vi "pll_proba_diag.vi"(0 "all rows":dbl[][](array[numeric])=array100002x3[300006 elements] format="%0.5f", 1 "Second":bool, 5 "Resolution":dbl, 7 "t_ref":dbl[](array[numeric]), 9 "dt":dbl, 11 "Error In":errorcluster) -> (3 "average":dbl=2.3596690204414683, 4 "XY Graph":cluster{"all rows":dbl[], "all rows":dbl[]}[](graph), 6 "Waveform Graph":cluster{"f0":dbl, "df":dbl, "magnitude":dbl[]}(graph), 8 "time":dbl[](array[numeric]), 10 "Waveform Graph 2":cluster{"f0":dbl, "df":dbl, "magnitude":dbl[]}(graph), 13 "PLL_sine":dbl[](array[numeric]), 14 "PLL_cosine":dbl[](array[numeric]), 15 "Error Out":errorcluster)   [LabVIEW 2013]
uses:
  <vilib>/Utility/file.llb/Read From Spreadsheet File (DBL).vi
  <vilib>/Utility/file.llb/Write To Spreadsheet File (DBL).vi
  <vilib>/express/express analysis/Spectral/Block/exnSpectralBlock spectral measurements RMS poly.vi
  <vilib>/express/express analysis/Spectral/Block/exnSpectralBlock spectral measurements RMS WFM.vi
  <vilib>/express/express analysis/Spectral/XNode/ExpressSpectralMeasurementsBlockNode.xnode
panel:
  out "sin(x)":dbl[](array[numeric])
  out "Array":dbl[](array[numeric])
  out "file path (use dialog)":path=path "C:/Users/Orban Anges/Desktop/DIAG_Prog_v2/temp.txt"
  out "XY Graph 2":cluster{"all rows":dbl[], "all rows":dbl[]}[](graph)
  out "t_i-1":dbl
  out "t_i":dbl
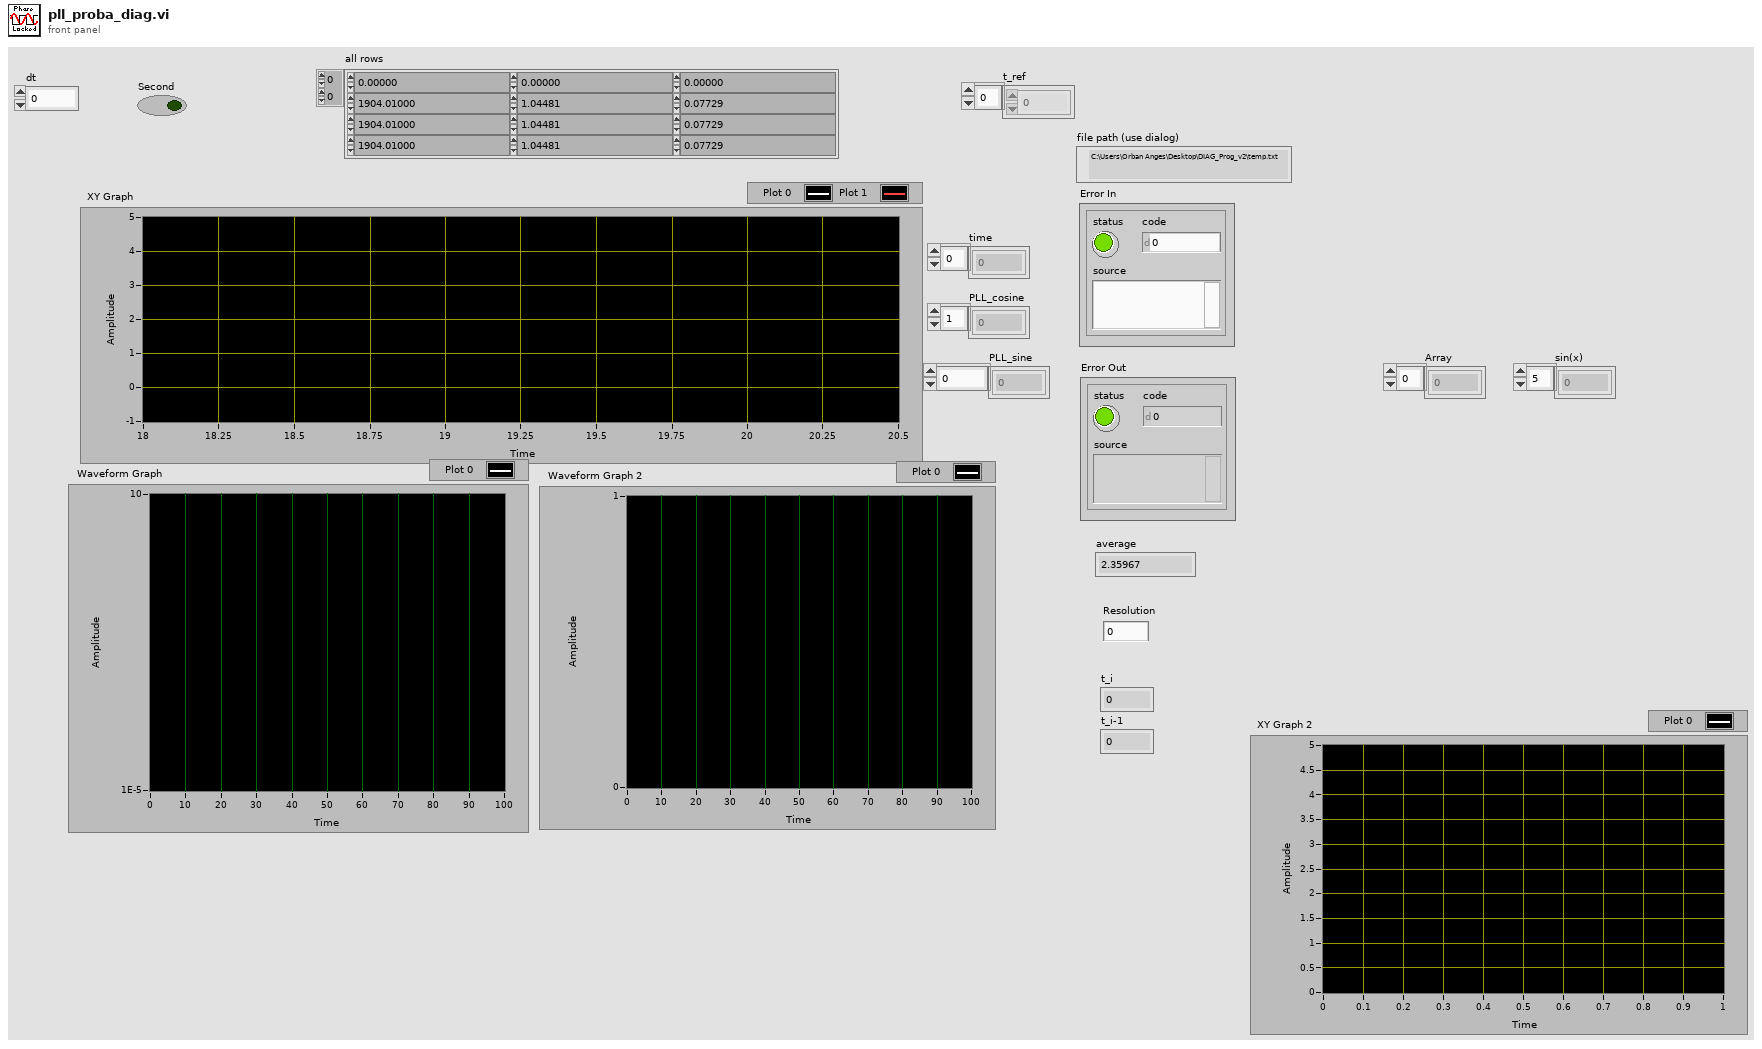
[diagram p1: front panel]
types:
  T1 = enum16{"open", "replace", "create", "open or create", "replace or create", "replace or create with confirmation"}
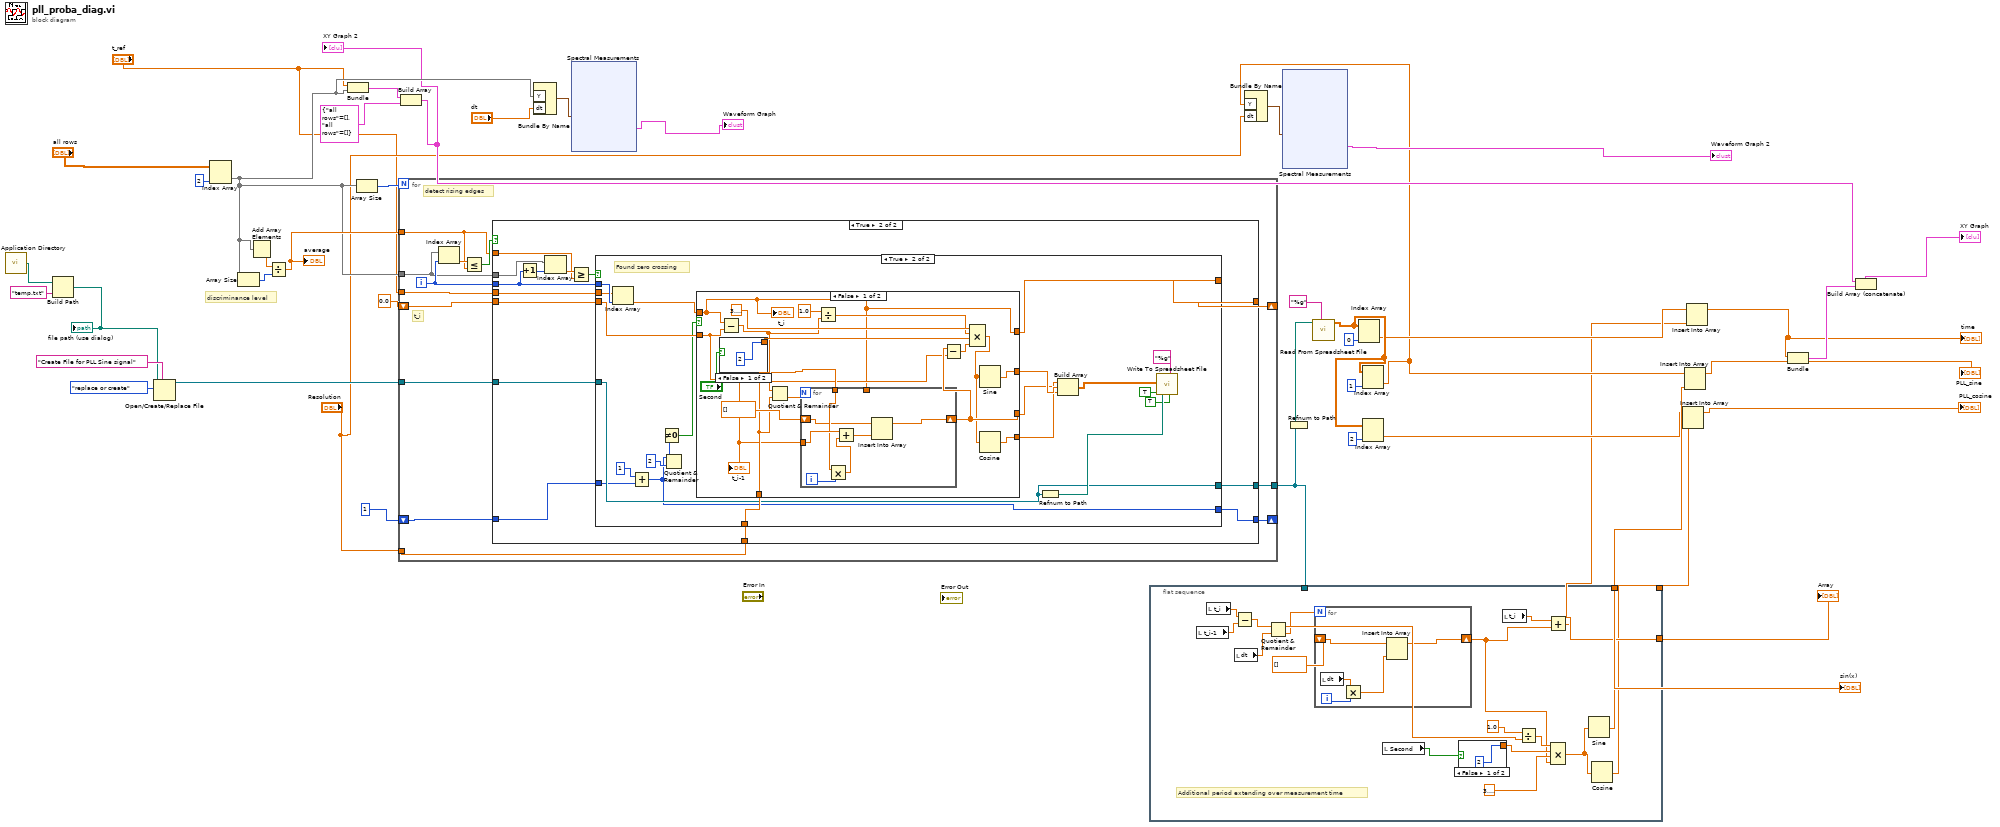
[diagram p0: block diagram]
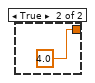
[diagram p2: hidden frame]
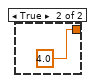
[diagram p5: hidden frame]
diagram:
  # "discriminance level"
  n1 = call <vilib>:"Application Directory.vi"() -> ("Application Directory"=w14:path)
  n2 = Build Path(base path=w14, name or relative path="temp.txt") -> (appended path=w12:path)
  "file path (use dialog)" <- w12
  n3 = Open/Create/Replace File(file path (use dialog)=w12, prompt="Create File for PLL Sine signal", operation (0:open)=T1."replace or create") -> (refnum out=w34:refnum<file>)  [unwired: 3 in, 2 out]
  n4 = Index Array(array="all rows", index (col)=2 ("disabled index (col)")) -> (element=w27:dbl[])  [unwired: 1 in]
  n5 = Array Size(array=w27) -> (size(s)=w40:i32)
  n6 = Add Array Elements(numeric array=w27) -> (sum=w41:dbl)
  n7 = Divide(x=w41, y=w40) -> (x/y=w39:dbl)
  "average" <- w39
  n8 = Bundle("t_ref"="t_ref", "all rows"=w27) -> (w21:cluster{"t_ref":dbl[], "all rows":dbl[]})  [unwired: 1 in]
  n9 = Array Size(array=w27) -> (size(s)=w38:i32)
  n10 = for {
    N: w38 -> [_]
    tunnel: w27 -> [w54]
    tunnel: w39 -> [w52]
    tunnel: "t_ref" -> [w51]
    shift-right: [w50] -> _
    shift-left: 0.0 -> [w44]
    tunnel: "Resolution" -> [w49]
    tunnel: w34 -> [w48]
    tunnel: [w47] -> w1
    shift-right: [w45] -> _
    shift-left: 1 -> [w46]
    i -> [w55]
    # "t_i"
    # "detect rising edges"
    n11 = Index Array(array=w54, index=w55) -> (element=w53:dbl)
    n12 = Less Or Equal?(x=w53, y=w52) -> (x <= y?=w56:bool)
    n13 = case shown="True" w56 {
      tunnel: w55 -> [_ w67]
      tunnel: w54 -> [_ w73]
      tunnel: w52 -> [_ w69]
      tunnel: w51 -> [_ w68]
      tunnel: [w59 w66] -> w50
      tunnel: w44 -> [w59 w60]
      tunnel: w49 -> [_ w65]
      tunnel: w48 -> [w58 w64]
      tunnel: [w58 w63] -> w47
      tunnel: w46 -> [w57 w62]
      tunnel: [w57 w61] -> w45
      frame False {
      }
      frame True {
        n14 = Increment(x=w67) -> (x+1=w72:i32)
        n15 = Index Array(array=w73, index=w72) -> (element=w70:dbl)
        n16 = Greater Or Equal?(x=w70, y=w69) -> (x >= y?=w71:bool)
        n17 = case shown="True" w71 {
          tunnel: w68 -> [_ w96]
          tunnel: w67 -> [_ w97]
          tunnel: [w76 w79] -> w66
          tunnel: w60 -> [w76 w94]
          tunnel: w65 -> [_ w95]
          tunnel: w64 -> [w75 w91]
          tunnel: [w75 w91] -> w63
          tunnel: w62 -> [w74 w83]
          tunnel: [w74 w78] -> w61
          frame False {
          }
          frame True {
            # "Found zero crossing"
            n18 = Index Array(array=w96, index=w97) -> (element=w77:dbl)
            n19 = Add(x=1, y=w83) -> (x+y=w78:i32)
            n20 = Quotient & Remainder(x=w78, y=2) -> (x-y*floor(x/y)=w81:i32)  [unwired: 1 out]
            n21 = Not Equal To 0?(x=w81) -> (x != 0?=w80:bool)
            n22 = case shown="False" w80 {
              tunnel: w94 -> [w99 w123]
              tunnel: w77 -> [w98 _]
              tunnel: w95 -> [w104 _]
              tunnel: [w107 _] -> w86
              tunnel: [w111 _] -> w88
              tunnel: [w101 _] -> w85
              tunnel: [w98 w123] -> w79
              frame False {
                n23 = case shown="False" "Second" {
                  tunnel: [2 4.0 ("value")] -> w112
                  frame False {
                  }
                  frame True {
                  }
                }
                n24 = Subtract(x=w98, y=w99) -> (x-y=w105:dbl)
                n25 = Quotient & Remainder(x=w105, y=w104) -> (floor(x/y)=w103:dbl)  [unwired: 1 out]
                n26 = for {
                  N: w103 -> [_]
                  tunnel: w104 -> [w120]
                  tunnel: w99 -> [w121]
                  tunnel: w98 -> [_]
                  shift-right: [w122] -> w107
                  shift-left: dbl[] [] -> [w116]
                  i -> [w118]
                  n27 = Multiply(x=w120, y=w118) -> (x*y=w119:dbl)
                  n28 = Add(x=w121, y=w119) -> (x+y=w117:dbl)
                  n29 = Insert Into Array(array=w116, new element=w117) -> (w122:dbl[])  [unwired: 1 in]
                }
                n30 = Divide(x=1.0, y=w105) -> (x/y=w109:dbl)
                n31 = Subtract(x=w107, y=w99) -> (x-y=w106:dbl[])
                n32 = Compound Arithmetic op=MULTIPLY(3.141592653589793, w109, w112, w106) -> (w102:dbl[])
                n33 = Sine(x=w102) -> (sin(x)=w111:dbl[])
                n34 = Cosine(x=w102) -> (cos(x)=w101:dbl[])
                "t_i-1" <- w99
                "t_i" <- w98
              }
              frame True {
              }
            }
            n35 = Refnum to Path(1:w91) -> (0:w92:path)
            n36 = Build Array(w86, w88, w85) -> (w87:dbl[][])
            n37 = call-poly <vilib>:"Write To Spreadsheet File.vi"("transpose? (no:F)"=TRUE, "format (%.3f)"="%g", "append to file? (new file:F)"=TRUE, "2D data"=w87, "file path (dialog if empty)"=w92) -> ()  [unwired: 3 in, 1 out]
          }
        }
      }
    }
  }
  n38 = Build Array(w21, cluster{"all rows":dbl[], "all rows":dbl[]} {"all rows"=[], "all rows"=[]} ("element")) -> (w19:cluster{"all rows":dbl[], "all rows":dbl[]}[])
  "XY Graph 2" <- w19
  n39 = Bundle By Name("Y"=w27, "dt"="dt") -> (w28:waveform(dbl))  [unwired: 1 in]
  n40 = xnode "Spectral Measurements"("Signals"=w28) -> ("FFT - (RMS)"=→"Waveform Graph":cluster{"f0":dbl, "df":dbl, "magnitude":dbl[]})  [unwired: 1 in, 2 out]
  n41 = flat-sequence {
    tunnel: [w131] -> w7
    tunnel: [w130] -> w5
    tunnel: [w126] -> w2
    tunnel: w1 -> [_]
    frame #0 {
      # "Additional period extending over measurement time"
      n42 = local read "t_i-1"() -> (w124:dbl)
      n43 = local read "t_i"() -> (w125:dbl)
      n44 = Subtract(x=w125, y=w124) -> (x-y=w138:dbl)
      n45 = local read "dt"() -> (w140:dbl)
      n46 = Quotient & Remainder(x=w138, y=w140) -> (floor(x/y)=w129:dbl)  [unwired: 1 out]
      n47 = for {
        N: w129 -> [_]
        shift-right: [w147] -> w127
        shift-left: dbl[] [] -> [w145]
        i -> [w146]
        n48 = local read "dt"() -> (w144:dbl)
        n49 = Multiply(x=w144, y=w146) -> (x*y=w143:dbl)
        n50 = Insert Into Array(array=w145, new element=w143) -> (w147:dbl[])  [unwired: 1 in]
      }
      n51 = local read "Second"() -> (w139:bool)
      n52 = case shown="False" w139 {
        tunnel: [2 4.0 ("value")] -> w135
        frame False {
        }
        frame True {
        }
      }
      n53 = local read "t_i"() -> (w128:dbl)
      n54 = Divide(x=1.0, y=w138) -> (x/y=w136:dbl)
      n55 = Add(x=w128, y=w127) -> (x+y=w126:dbl[])
      n56 = Compound Arithmetic op=MULTIPLY(w136, w135, 3.141592653589793, w127) -> (w132:dbl[])
      n57 = Sine(x=w132) -> (sin(x)=w131:dbl[])
      n58 = Cosine(x=w132) -> (cos(x)=w130:dbl[])
    }
  }
  n59 = Refnum to Path(1:w1) -> (0:w33:path)
  n60 = call-poly <vilib>:"Read From Spreadsheet File.vi"("format (%.3f)"="%g", "file path (dialog if empty)"=w33) -> ("all rows"=w22:dbl[][])  [unwired: 5 in, 4 out]
  n61 = Index Array(array=w22, index (col)=0 ("disabled index (col)")) -> (element=w10:dbl[])  [unwired: 1 in]
  n62 = Index Array(array=w22, index (col)=1 ("disabled index (col)")) -> (element=w8:dbl[])  [unwired: 1 in]
  n63 = Bundle By Name("Y"=w8, "dt"="Resolution") -> (w25:waveform(dbl))  [unwired: 1 in]
  n64 = xnode "Spectral Measurements"("Signals"=w25) -> ("FFT - (RMS)"=→"Waveform Graph 2":cluster{"f0":dbl, "df":dbl, "magnitude":dbl[]})  [unwired: 1 in, 2 out]
  n65 = Index Array(array=w22, index (col)=2) -> (element=w6:dbl[])  [unwired: 1 in]
  n66 = Insert Into Array(array=w6, new element=w5) -> (→"PLL_cosine":dbl[])  [unwired: 1 in]
  n67 = Insert Into Array(array=w8, new element=w7) -> (w3:dbl[])  [unwired: 1 in]
  "PLL_sine" <- w3
  n68 = Insert Into Array(array=w10, new element=w2) -> (w9:dbl[])  [unwired: 1 in]
  "time" <- w9
  n69 = Bundle("all rows"=w9, "all rows"=w3) -> (w29:cluster{"all rows":dbl[], "all rows":dbl[]})  [unwired: 1 in]
  n70 = Build Array (concatenate)(w19, w29) -> (→"XY Graph":cluster{"all rows":dbl[], "all rows":dbl[]}[])
  "Array" <- w2
  "sin(x)" <- w7
